vi "DownloadRun.vi"(11 "Data In":T1={"VISA Refnum in"="", "All Code"="Hi"}) -> (0 "error out":errorcluster, 3 "VISA Refnum out":refnum<visa-resource-name>)   [LabVIEW 2016]
panel:
  out "key":string
  in  "Ctrl B":bool
  in  "Ctrl D":bool
  in  "Ctrl C":bool
  out "Console":string
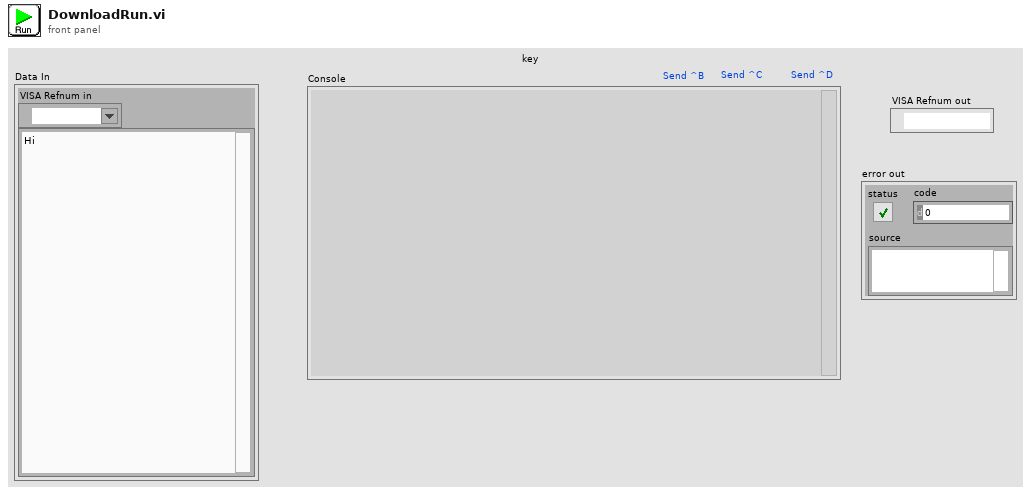
[diagram p1: front panel]
types:
  T1 = cluster{"VISA Refnum in":refnum<visa-resource-name>, "All Code":string}
  T2 = typedef "eventvkey.ctl" = enum16{"ASCII", "Enter", "Return", "Shift", "Ctrl", "Alt", "Cmd", "Opt", "Caps", "NumLock", "Clear", "Break", "Up", "Down", "Left", "Right", "Insert", "Delete", "Home", "End", "PageUp", "PageDown", "Escape", "Help", "Pause", "ScrollLock", "F1", "F2", "F3", "F4", "F5", "F6", "F7", "F8", "F9", "F10", "F11", "F12", "F13", "F14", "F15", "F16", "F17", "F18", "F19", "F20", "F21", "F22", "F23", "F24", "Play", "VolumeUp", "VolumeDown", "Mute", "Two Byte Char"}
  T3 = cluster{"Shift":bool, "Ctrl":bool, "Alt":bool, "Cmd":bool, "Opt":bool}
  T4 = cluster{"Char":i16, "VKey":T2, "ScanCode":i16, "Mods":cluster{"Num Pad":bool, "Menu Key":bool}, "PlatMods":cluster{"Shift":bool, "Ctrl":bool, "Alt":bool, "Cmd":bool, "Opt":bool}, "FocusObj":refnum<vi>}
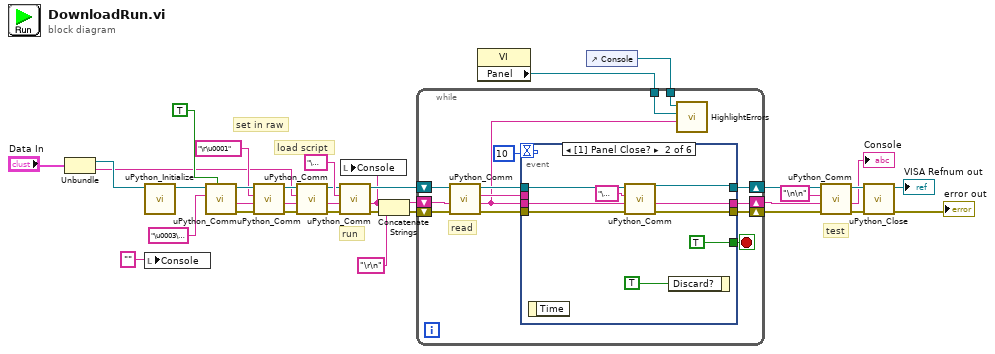
[diagram p0: block diagram]
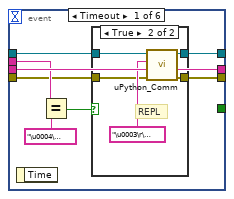
[diagram p2: hidden frame]
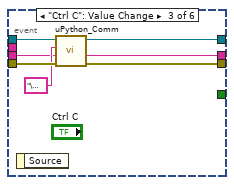
[diagram p4: hidden frame]
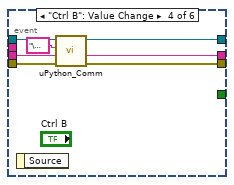
[diagram p5: hidden frame]
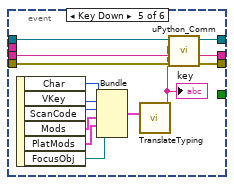
[diagram p6: hidden frame]
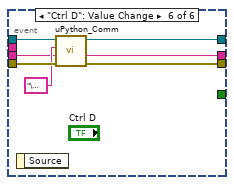
[diagram p7: hidden frame]
diagram:
  # "test"
  # "run"
  # "load script"
  # "set in raw"
  n1 = Unbundle("Data In") -> ("VISA Refnum in"=w11:refnum<visa-resource-name>, "All Code"=w10:string)
  n2 = call "uPython_Initialize.vi"("VISA Refnum in"=w11) -> ("VISA Refnum out"=w33:refnum<visa-resource-name>)  [unwired: 9 in, 1 out]
  n3 = local write "Console"("" ("Console")) -> ()
  n4 = call "uPython_Comm.vi"("Wait for Reply?"=TRUE, "Script"="\u0003\u0003", "VISA Refnum in"=w33) -> ("error out"=w30:errorcluster, "Console Out"=w28:string, "VISA out"=w31:refnum<visa-resource-name>)  [unwired: 4 in, 2 out]
  n5 = call "uPython_Comm.vi"("error in (no error)"=w30, "Console In"=w28, "Script"="\r\u0001", "VISA Refnum in"=w31) -> ("error out"=w22:errorcluster, "Console Out"=w21:string, "VISA out"=w23:refnum<visa-resource-name>)  [unwired: 3 in, 2 out]
  n6 = call "uPython_Comm.vi"("error in (no error)"=w22, "Console In"=w21, "Script"=w10, "VISA Refnum in"=w23) -> ("error out"=w18:errorcluster, "Console Out"=w16:string, "VISA out"=w19:refnum<visa-resource-name>)  [unwired: 3 in, 2 out]
  n7 = call "uPython_Comm.vi"("error in (no error)"=w18, "Console In"=w16, "Script"="\u0004", "VISA Refnum in"=w19) -> ("error out"=w15:errorcluster, "Console Out"=w1:string, "VISA out"=w14:refnum<visa-resource-name>)  [unwired: 3 in, 2 out]
  n8 = local write "Console"(w1) -> ()
  n9 = Concatenate Strings(w1, "\r\n" ("Script")) -> (w12:string)
  n10 = property class="VI"() -> ("Panel"=w4:refnum<vi>)  [unwired: 2 in, 2 out]
  n11 = control-ref of="Console"() -> (w3:refnum<vi>)
  n12 = while {
    shift-right: [w39] -> w6
    shift-left: w15 -> [w48]
    shift-right: [w40] -> w7
    shift-left: w14 -> [w47]
    shift-right: [w41] -> w5
    shift-left: w12 -> [w46]
    tunnel: w4 -> [w36]
    tunnel: w3 -> [w35]
    stop <- w44 stop-if-true
    # "read"
    n13 = call "uPython_Comm.vi"("error in (no error)"=w48, "Console In"=w46, "VISA Refnum in"=w47) -> ("error out"=w42:errorcluster, "Console Out"=w37:string, "Buffer"=w38:string, "VISA out"=w43:refnum<visa-resource-name>)  [unwired: 4 in, 1 out]
    n14 = event shown="[1] Panel Close?" {
      selector: _ -> [_ _ _ _ _ _]
      dyn-events: _ -> [_ _ _ _ _ _]
      timeout: 10 -> [_ _ _ _ _ _]
      tunnel: [_ TRUE _ _ _ _] -> w44
      tunnel: w43 -> [w52 w69 w79 w86 w100 w107]
      tunnel: w42 -> [w50 w65 w78 w85 w99 w106]
      tunnel: w37 -> [w56 w67 w74 w81 w96 w104]
      tunnel: [w56 w66 w75 w82 w97 w103] -> w41
      tunnel: [w51 w68 w76 w83 w98 w102] -> w40
      tunnel: [w49 w64 w73 w80 w95 w101] -> w39
      tunnel: w38 -> [w54 _ _ _ _ _]
      event Timeout {
        n15 = event-data() -> ()  [unwired: 1 in, 1 out]
        n16 = Equal?(x=w54, y="\u0004\u0004>" ("Script")) -> (x = y?=w53:bool)
        n17 = case shown="True" w53 {
          tunnel: w52 -> [w58 w62]
          tunnel: [w58 w61] -> w51
          tunnel: w50 -> [w57 w60]
          tunnel: [w57 w59] -> w49
          frame False {
          }
          frame True {
            # "REPL"
            n18 = call "uPython_Comm.vi"("error in (no error)"=w60, "Script"="\u0003\r\u0002", "VISA Refnum in"=w62) -> ("error out"=w59:errorcluster, "VISA out"=w61:refnum<visa-resource-name>)  [unwired: 4 in, 3 out]
          }
        }
      }
      event Panel Close? {
        n19 = event-data() -> ()  [unwired: 1 in, 1 out]
        n20 = call "uPython_Comm.vi"("error in (no error)"=w65, "Console In"=w67, "Script"="\u0002", "VISA Refnum in"=w69) -> ("error out"=w64:errorcluster, "Console Out"=w66:string, "VISA out"=w68:refnum<visa-resource-name>)  [unwired: 3 in, 2 out]
        n21 = event-data("Discard?"=TRUE) -> ()  [unwired: 1 in, 1 out]
      }
      event "Ctrl C": Value Change {
        n22 = event-data() -> ()  [unwired: 1 in, 1 out]
        n23 = call "uPython_Comm.vi"("error in (no error)"=w78, "Console In"=w74, "Script"="\u0003", "VISA Refnum in"=w79) -> ("error out"=w73:errorcluster, "Console Out"=w75:string, "VISA out"=w76:refnum<visa-resource-name>)  [unwired: 3 in, 2 out]
      }
      event "Ctrl B": Value Change {
        n24 = event-data() -> ()  [unwired: 1 in, 1 out]
        n25 = call "uPython_Comm.vi"("error in (no error)"=w85, "Console In"=w81, "Script"="\u0002", "VISA Refnum in"=w86) -> ("error out"=w80:errorcluster, "Console Out"=w82:string, "VISA out"=w83:refnum<visa-resource-name>)  [unwired: 3 in, 2 out]
      }
      event Key Down {
        n26 = event-data() -> ("Char"=w94:i16, "VKey"=w93:T2, "ScanCode"=w92:i16, "Mods"=w91:cluster{"Num Pad":bool, "Menu Key":bool}, "PlatMods"=w90:T3, "FocusObj"=w89:refnum<vi>)  [unwired: 1 in]
        n27 = Bundle("Char"=w94, "VKey"=w93, "ScanCode"=w92, "Mods"=w91, "PlatMods"=w90, "FocusObj"=w89) -> (w88:T4)  [unwired: 1 in]
        n28 = call "TranslateTyping.vi"("Cluster"=w88) -> ("key"=w87:string)  [unwired: 8 in, 2 out]
        "key" <- w87
        n29 = call "uPython_Comm.vi"("error in (no error)"=w99, "Console In"=w96, "Script"=w87, "VISA Refnum in"=w100) -> ("error out"=w95:errorcluster, "Console Out"=w97:string, "VISA out"=w98:refnum<visa-resource-name>)  [unwired: 3 in, 2 out]
      }
      event "Ctrl D": Value Change {
        n30 = event-data() -> ()  [unwired: 1 in, 1 out]
        n31 = call "uPython_Comm.vi"("error in (no error)"=w106, "Console In"=w104, "Script"="\u0004", "VISA Refnum in"=w107) -> ("error out"=w101:errorcluster, "Console Out"=w103:string, "VISA out"=w102:refnum<visa-resource-name>)  [unwired: 3 in, 2 out]
      }
    }
    n32 = call "HighlightErrors.vi"("String"=w37, "Front Panel"=w36, "Console"=w35) -> ()  [unwired: 9 in]
  }
  n33 = call "uPython_Comm.vi"("error in (no error)"=w6, "Console In"=w5, "Script"="\n\n", "VISA Refnum in"=w7) -> ("error out"=w27:errorcluster, "Console Out"=→"Console":string, "VISA out"=w26:refnum<visa-resource-name>)  [unwired: 3 in, 2 out]
  n34 = call "uPython_Close.vi"("error in"=w27, "VISA  in"=w26) -> ("error out"=→"error out":errorcluster, "VISA  out"=→"VISA Refnum out":refnum<visa-resource-name>)  [unwired: 8 in]
